vi "DMM_PickBaseline.vi"(0 "InputPick":refnum<data-value>, 1 "SignalRef":refnum<data-value>, 3 "Input DMMP":refnum<class "DMMP.lvclass">) -> (2 "Reference":dbl, 4 "State":string="Baseline", 5 "Output DMMP":refnum<class "DMMP.lvclass">)   [LabVIEW 2014]
uses:
  DMMP.lvclass
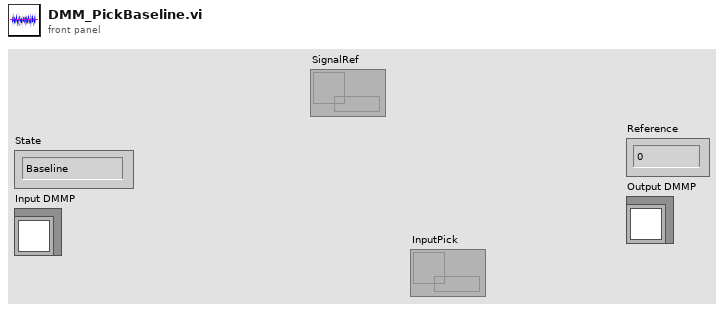
[diagram p1: front panel]
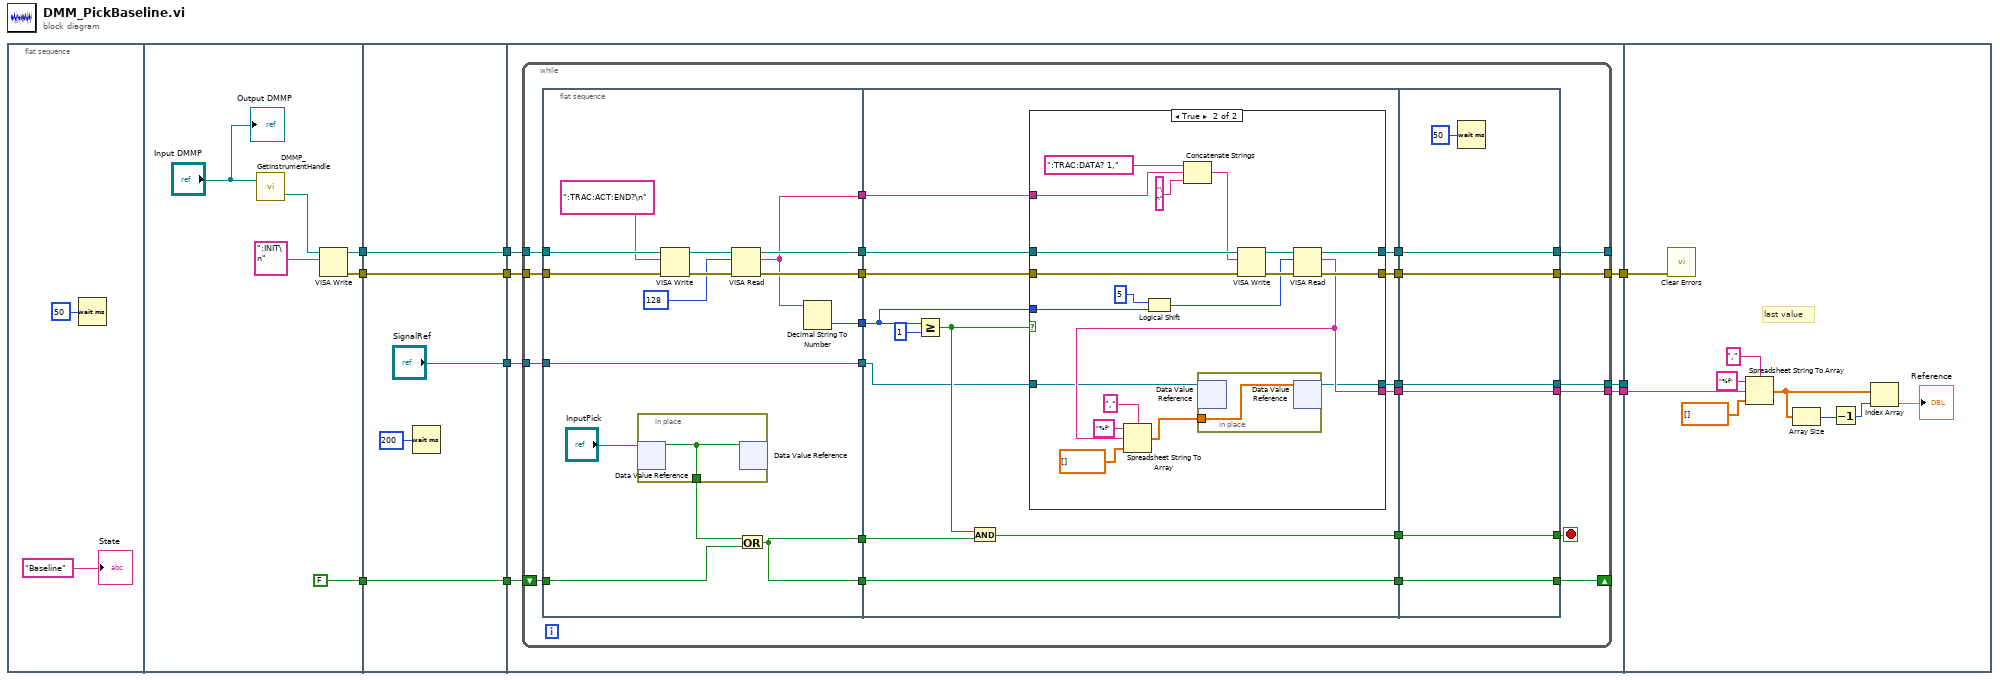
[diagram p0: block diagram]
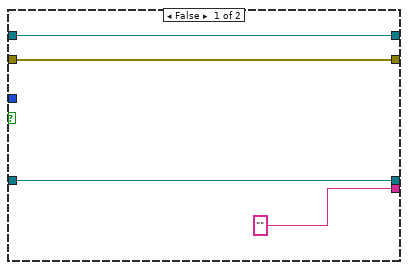
[diagram p2: hidden frame]
diagram:
  n1 = flat-sequence {
    tunnel: [w15] -> w8
    tunnel: [w14] -> w6
    tunnel: [FALSE] -> w4
    tunnel: w8 -> [w23]
    tunnel: [w23] -> w7
    tunnel: w6 -> [w22]
    tunnel: [w22] -> w5
    tunnel: w4 -> [w21]
    tunnel: [w21] -> w3
    tunnel: ["SignalRef"] -> w2
    tunnel: w7 -> [w30]
    tunnel: w5 -> [w29]
    tunnel: w3 -> [w28]
    tunnel: [w27] -> w10
    tunnel: [w26] -> w9
    tunnel: w2 -> [w25]
    tunnel: [w24] -> w1
    tunnel: w10 -> [w123]
    tunnel: w9 -> [w116]
    tunnel: w1 -> [_]
    frame #0 {
      n2 = Wait (ms)(milliseconds to wait=u32 50) -> ()  [unwired: 1 out]
      "State" <- "Baseline"
    }
    frame #1 {
      n3 = call "DMMP_GetInstrumentHandle.vi"("Input DMMP"="Input DMMP") -> ("DMM Serial Port"=w17:refnum<visa-resource-name>)  [unwired: 1 in, 1 out]
      n4 = VISA Write(VISA resource name=w17, write buffer=":INIT\n") -> (VISA resource name out=w15:refnum<visa-resource-name>, error out=w14:errorcluster)  [unwired: 1 in, 1 out]
      "Output DMMP" <- "Input DMMP"
    }
    frame #2 {
      n5 = Wait (ms)(milliseconds to wait=u32 200) -> ()  [unwired: 1 out]
    }
    frame #3 {
      n6 = while {
        tunnel: w30 -> [w53]
        tunnel: w29 -> [w52]
        shift-right: [w41] -> _
        shift-left: w28 -> [w44]
        tunnel: [w37] -> w27
        tunnel: [w36] -> _
        tunnel: [w35] -> w26
        tunnel: w25 -> [w33]
        tunnel: [w31] -> w24
        stop <- w45 stop-if-true
        n7 = flat-sequence {
          tunnel: w53 -> [w68]
          tunnel: w52 -> [w64]
          tunnel: [w62] -> w51
          tunnel: [w61] -> w50
          tunnel: [w60] -> w49
          tunnel: [w57] -> w48
          tunnel: [w59] -> w47
          tunnel: w44 -> [w58]
          tunnel: [w57] -> w42
          tunnel: [w54] -> w34
          tunnel: w33 -> [w54]
          tunnel: w51 -> [w80]
          tunnel: w50 -> [w79]
          tunnel: w49 -> [w77]
          tunnel: w48 -> [w82]
          tunnel: w47 -> [w78]
          tunnel: [w76] -> w46
          tunnel: [w75] -> w43
          tunnel: w42 -> [w75]
          tunnel: [w74] -> w40
          tunnel: [w73] -> w39
          tunnel: [w72] -> w38
          tunnel: w34 -> [w71]
          tunnel: [w70] -> w32
          tunnel: w46 -> [w114]
          tunnel: [w114] -> w45
          tunnel: w43 -> [w113]
          tunnel: [w113] -> w41
          tunnel: w40 -> [w111]
          tunnel: w39 -> [w110]
          tunnel: w38 -> [w112]
          tunnel: [w112] -> w37
          tunnel: [w111] -> w36
          tunnel: [w110] -> w35
          tunnel: w32 -> [w109]
          tunnel: [w109] -> w31
          frame #0 {
            n8 = in-place {
              in-place-border: [w69] -> w55
              n9 = in-place-dvr #1("InputPick") -> (w69:bool)  [unwired: 1 out]
              n10 = in-place-dvr #1(w69) -> ()  [unwired: 2 out]
            }
            n11 = VISA Write(VISA resource name=w68, write buffer=":TRAC:ACT:END?\n", error in (no error)=w64) -> (VISA resource name out=w66:refnum<visa-resource-name>, error out=w65:errorcluster)  [unwired: 1 out]
            n12 = VISA Read(VISA resource name=w66, byte count=u32 128, error in (no error)=w65) -> (VISA resource name out=w62:refnum<visa-resource-name>, read buffer=w59:string, error out=w61:errorcluster)  [unwired: 1 out]
            n13 = Or(x=w55, y=w58) -> (x .or. y?=w57:bool)
            n14 = Decimal String To Number(string=w59) -> (number=w60:i32)  [unwired: 2 in, 1 out]
          }
          frame #1 {
            n15 = Greater Or Equal?(x=w77, y=1) -> (x >= y?=w81:bool)
            n16 = And(x=w81, y=w82) -> (x .and. y?=w76:bool)
            n17 = case shown="True" w81 {
              tunnel: w80 -> [w87 w107]
              tunnel: w79 -> [w86 w106]
              tunnel: w78 -> [_ w104]
              tunnel: w77 -> [_ w99]
              tunnel: [w87 w96] -> w74
              tunnel: [w86 w95] -> w73
              tunnel: ["" ("read buffer") w91] -> w72
              tunnel: w71 -> [w84 w90]
              tunnel: [w84 w88] -> w70
              frame False {
              }
              frame True {
                n18 = Logical Shift(y=5, x=w99) -> (x << y=w97:i32)
                n19 = Concatenate Strings(":TRAC:DATA? 1," ("string"), w104, "\n" ("string")) -> (w102:string)
                n20 = VISA Write(VISA resource name=w107, write buffer=w102, error in (no error)=w106) -> (VISA resource name out=w101:refnum<visa-resource-name>, error out=w100:errorcluster)  [unwired: 1 out]
                n21 = VISA Read(VISA resource name=w101, byte count=w97, error in (no error)=w100) -> (VISA resource name out=w96:refnum<visa-resource-name>, read buffer=w91:string, error out=w95:errorcluster)  [unwired: 1 out]
                n22 = Spreadsheet String To Array(delimiter (Tab)=",", format string="%f", spreadsheet string=w91, array type (2D Dbl)=dbl[] []) -> (array=w89:dbl[])
                n23 = in-place {
                  in-place-border: w89 -> [w108]
                  n24 = in-place-dvr #2(w90) -> ()  [unwired: 2 out]
                  n25 = in-place-dvr #2(w108) -> (w88:refnum<data-value>)  [unwired: 1 out]
                }
              }
            }
          }
          frame #2 {
            n26 = Wait (ms)(milliseconds to wait=u32 50) -> ()  [unwired: 1 out]
          }
        }
      }
    }
    frame #4 {
      # "last value"
      n27 = call <vilib>:"Clear Errors.vi"("error in (no error)"=w116) -> ()  [unwired: 5 in, 2 out]
      n28 = Spreadsheet String To Array(delimiter (Tab)=",", format string="%f", spreadsheet string=w123, array type (2D Dbl)=dbl[] []) -> (array=w119:dbl[])
      n29 = Array Size(array=w119) -> (size(s)=w118:i32)
      n30 = Decrement(x=w118) -> (x-1=w117:i32)
      n31 = Index Array(array=w119, index=w117) -> (element=→"Reference":dbl)
    }
  }
